vi "Test.vi"() -> ()   [LabVIEW 2011]
uses:
  Simple Error Out.xctl
panel:
  in  "error in (no error) 3":errorcluster={"status"=TRUE, "code"=7, "source"="Test Source"}
  out "Simple Error Out 3":errorcluster(xcontrol)
  in  "error in (no error) 2":errorcluster={"status"=TRUE, "code"=7, "source"="Test Source"}
  out "Simple Error Out 2":errorcluster(xcontrol)
  in  "stop":bool
  in  "error in (no error)":errorcluster={"status"=TRUE, "code"=7, "source"="Test Source"}
  out "Simple Error Out":errorcluster(xcontrol)
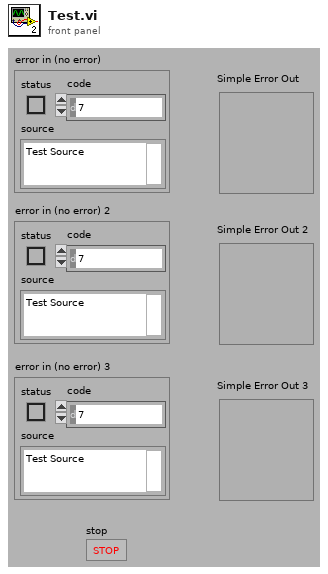
[diagram p1: front panel]
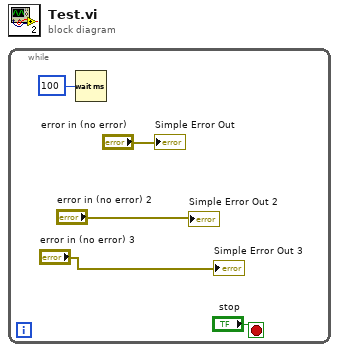
[diagram p0: block diagram]
diagram:
  n1 = while {
    stop <- "stop" stop-if-true
    n2 = Wait (ms)(milliseconds to wait=u32 100 ("millisecond timer value")) -> ()  [unwired: 1 out]
    "Simple Error Out" <- "error in (no error)"
    "Simple Error Out 2" <- "error in (no error) 2"
    "Simple Error Out 3" <- "error in (no error) 3"
  }
